vi "test Block Upload Sim.vi"(11 "Test Case In":refnum<class "Tests SDO Manager.lvclass">) -> (0 "error out":errorcluster, 3 "Test Case Out":refnum<class "Tests SDO Manager.lvclass">)   [LabVIEW 2020, in "Tests SDO Manager.lvclass"]
uses:
  Tests SDO Manager.lvclass
  source/Logging/Logger/Logger.lvclass
  Simulated CANopen Node/Simulated CANopen Node.lvclass
  <vilib>/ActorFramework/Stop Msg/Stop Msg.lvclass
  HAL/Source/Interfaces/IMessage/IMessage.lvclass
  Tests SDO Manager.lvclass/Tests SDO Manager.ctl
  4993e8ee-a06a-463a-9684-69129f64d5ce.vi
  source/SDO Manager/SDO Manager/SDO Manager/SDO Manager.lvclass
  source/Logging/Log Level.vi
  source/Logging/CANopen Logging.lvlib
  <vilib>/ActorFramework/Actor/Actor.lvclass
  source/SDO Manager/SDO Manager/SDO Transfer/SDO abort code.ctl
  source/SDO Manager/SDO Manager/SDO Transfer/SDO Transfer.lvclass
  source/Typedefs/SDO Result.ctl
panel:
  out "SDO Result":T1={"Success"=FALSE, "SDO abort code"={"Null"=TRUE, "Value"=84082688}, "Data"={"Null"=TRUE, "Data"=[]}} {"SDO abort code"."Value" items=["Toggle bit not allowed"=84082688, "SDO protocol timed out"=84148224, "Client/server command specifier not valid or unknown"=84148225, "Invalid block size (block mode only)"=84148226, "Invalid sequence number (block mode only)"=84148227, "CRC error (block mode only)"=84148228, "Out of memory"=84148229, "Attempt to read a write only object"=100728833, "Attempt to write a read only object"=100728834, "Object does not exist in the object dictionary"=100794368, "Object cannot be mapped to the PDO"=100925505, "The number and length of the objects to be mapped would exceed PDO length"=100925506, "General parameter incompatibility reason"=100925507, "General internal incompatibility in the device"=100925511, "Access failed due to an hardware error"=101056512, "Data type does not match, length of service parameter does not match"=101122064, "Data type does not match, length of service parameter too high"=101122066, "Data type does not match, length of service parameter too low"=101122067, "Sub-index does not exist"=101253137, "Invalid value for parameter (download only)"=101253168, "Value of parameter written too high (download only)"=101253169, "Value of parameter written too low (download only)"=101253170, "Maximum value is less than minimum value"=101253174, "Resource not available: SDO connection"=101318691, "General error"=134217728, "Data cannot be transferred or stored to the application"=134217760, "Data cannot be transferred or stored to the application because of local control"=134217761, "Data cannot be transferred or stored to the application because of the present device stable"=134217762, "Object dictionary dynamic generation fails or no object dictionary is present (e.g. object dictionary is generated from file and generation fails because of an file error)"=134217763, "No data available"=134217764]; "Data"."Data" format="%02x"}
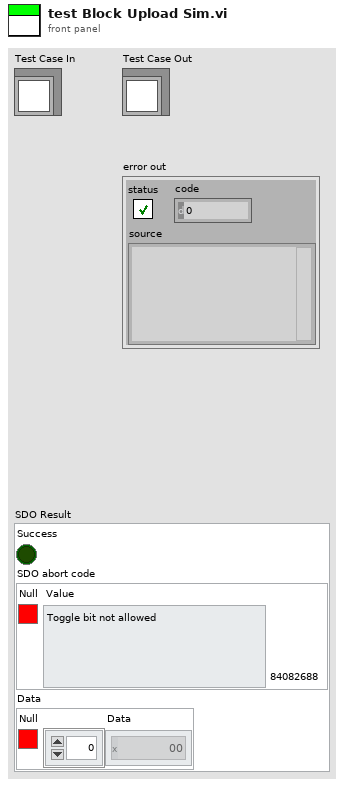
[diagram p1: front panel]
types:
  T1 = typedef "CANopen.lvlib/SDO Manager.lvlib/SDO Transfer.lvclass/SDO Result.ctl" = cluster{"Success":bool, "SDO abort code":cluster{"Null":bool, "Value":T2}, "Data":cluster{"Null":bool, "Data":u8[]}}
  T2 = typedef "CANopen.lvlib/SDO Manager.lvlib/SDO Transfer.lvclass/SDO abort code.ctl" = u32
  T3 = cluster{"Node-ID":u8, "Multiplexer":cluster{"Index":u16, "Sub-Index":u8}, "Data":u8[]}
  T4 = enum16{"Error", "Warn", "Info", "Debug", "Trace"}
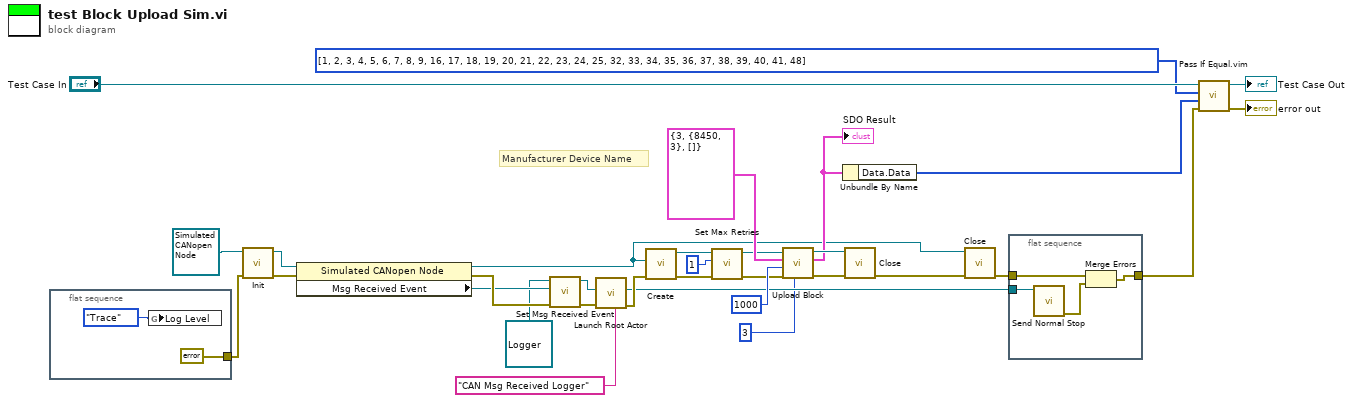
[diagram p0: block diagram]
diagram:
  # "Manufacturer Device Name"
  n1 = flat-sequence {
    tunnel: [errorcluster {"status"=FALSE, "code"=0, "source"=""} ("error constant")] -> w6
    frame #0 {
      n2 = global write "Log Level.vi" "Log Level"(T4."Trace" ("Log Level")) -> ()
    }
  }
  n3 = call-dynamic "Init.vi"("error in"=w6, "Simulated CANopen Node in"=refnum<class "Simulated CANopen Node.lvclass"> refnum ("Simulated CANopen Node.lvclass")) -> ("error out"=w21:errorcluster, "Simulated CANopen Node out"=w20:refnum<class "Simulated CANopen Node.lvclass">)  [unwired: 8 in]
  n4 = property class="Simulated CANopen Node"(reference=w20, error in=w21) -> (reference out=w5:refnum<class "Simulated CANopen Node.lvclass">, error out=w19:errorcluster, "Msg Received Event"=w18:refnum<user-event>)
  n5 = call "Set Msg Received Event.vi"("error in"=w19, "Msg Received Event"=w18, "Logger in"=refnum<class "Logger.lvclass"> refnum) -> ("error out"=w23:errorcluster, "Logger out"=w22:refnum<class "Logger.lvclass">)  [unwired: 7 in]
  n6 = call <vilib>:"Launch Root Actor.vi"("Debug Alias"="CAN Msg Received Logger", "error in (no error)"=w23, "Actor"=w22) -> ("error out"=w17:errorcluster, "Actor's Enqueuer"=w14:refnum<class "Message Enqueuer.lvclass">)  [unwired: 7 in]
  n7 = call "Create.vi"("Error In"=w17, "ICommunicate"=w5) -> ("Error Out"=w12:errorcluster, "SDO Manager"=w11:refnum<class "SDO Manager.lvclass">)  [unwired: 8 in]
  n8 = call "Set Max Retries.vi"("error in"=w12, "Max Retries"=u8 1, "SDO Manager in"=w11) -> ("error out"=w9:errorcluster, "SDO Manager out"=w10:refnum<class "SDO Manager.lvclass">)  [unwired: 7 in]
  n9 = call "Upload Block.vi"("Block size"=u8 3 ("Blocksize"), "error in"=w9, "Retry Delay (ms)"=1000 ("Timeout"), "Parameters"=T3 {"Node-ID"=3, "Multiplexer"={"Index"=8450, "Sub-Index"=3}, "Data"=[]}, "SDO Manager in"=w10) -> ("error out"=w27:errorcluster, "SDO Result"=w24:T1, "SDO Manager out"=w26:refnum<class "SDO Manager.lvclass">)  [unwired: 4 in]
  "SDO Result" <- w24
  n10 = Unbundle By Name(w24) -> ("Data.Data"=w2:u8[])
  n11 = call "Close.vi"("Error In"=w27, "SDO Manager"=w26) -> ("Error Out"=w29:errorcluster)  [unwired: 8 in, 1 out]
  n12 = call-dynamic "Close.vi"("error in"=w29, "Simulated CANopen Node in"=w5) -> ("error out"=w15:errorcluster)  [unwired: 8 in, 1 out]
  n13 = flat-sequence {
    tunnel: w15 -> [w35]
    tunnel: w14 -> [w38]
    tunnel: [w36] -> w13
    frame #0 {
      n14 = call <vilib>:"Send Normal Stop.vi"("Message Enqueuer"=w38) -> ("error out"=w37:errorcluster)  [unwired: 10 in]
      n15 = Merge Errors(w35, w37) -> (w36:errorcluster)
    }
  }
  n16 = call "Pass If Equal.vim"("error in (no error)"=w13, "Actual"=w2, "Expected"=u8[] [1, 2, 3, 4, 5, 6, 7, 8, 9, 16, 17, 18, 19, 20, 21, 22, 23, 24, 25, 32, 33, 34, 35, 36, 37, 38, 39, 40, 41, 48], "LUnit Test Case In"="Test Case In") -> ("error out"=→"error out":errorcluster, "LUnit Test Case Out"=→"Test Case Out":refnum<class "Tests SDO Manager.lvclass">)  [unwired: 6 in]
